vi "tag select action.vi"(8 "engine":refnum<data-value>, 10 "CtlRef":refnum<vi>, 11 "module editor":refnum<data-value>) -> (0 "error out":errorcluster)   [LabVIEW 2013, in "My Awesome Control Modules editor node.lvclass"]
uses:
  My Awesome Control Modules editor node.lvclass
  <vilib>/NI/Tag Bus Data Framework/control module/configuration/control module configuration.lvclass
  <vilib>/NI/Tag Bus/tag/tag descriptor.lvclass
  <vilib>/NI/Configuration Framework/serializable configuration/NISE_CEF_serializable configuration.lvclass
  <vilib>/NI/Tag Bus Data Framework/Configuration Editor/Classes/Engine Parent/Engine Parent Editor Node.lvclass
  <vilib>/NI/Module Execution Interface/Engine Configuration/engine configuration.lvclass
  <vilib>/NI/Tag Bus Data Framework/control module/editor node/control module editor.lvclass
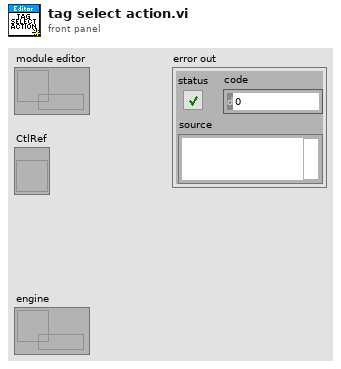
[diagram p1: front panel]
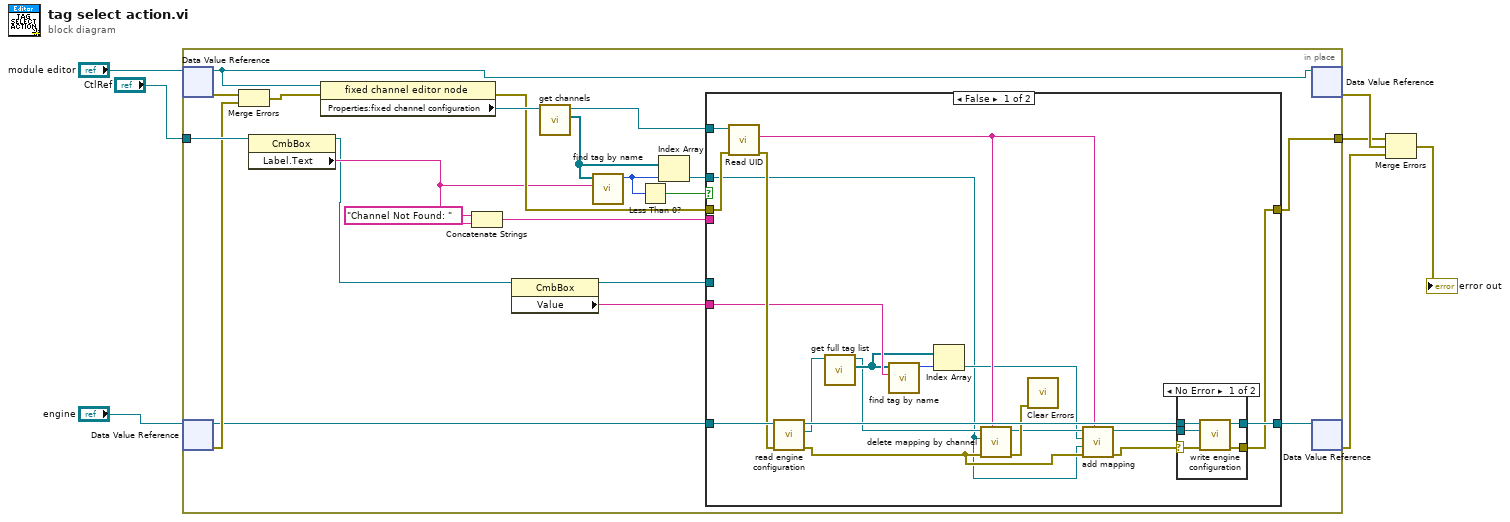
[diagram p0: block diagram]
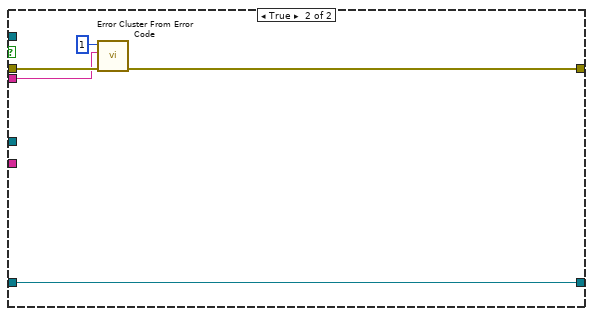
[diagram p3: hidden frame]
diagram:
  n1 = in-place {
    in-place-border: [w23] -> w2
    in-place-border: "CtlRef" -> [w21]
    n2 = in-place-dvr #1("module editor") -> (w13:refnum<class "control module editor.lvclass">, w28:errorcluster)
    n3 = in-place-dvr #2("engine") -> (w12:refnum<class "Engine Parent Editor Node.lvclass">, w15:errorcluster)
    n4 = Merge Errors(w28, w15) -> (w16:errorcluster)
    n5 = property class="CmbBox"(reference=w21) -> (reference out=w11:refnum<vi>, "Label.Text"=w20:string)  [unwired: 1 in, 1 out]
    n6 = property class="fixed channel editor node"(reference=w13, error in=w16) -> (error out=w22:errorcluster, "Properties:fixed channel configuration"=w27:refnum<class "control module configuration.lvclass">)  [unwired: 1 out]
    n7 = Concatenate Strings("Channel Not Found: " ("string"), w20) -> (w18:string)
    n8 = property class="CmbBox"(reference=w11) -> (reference out=w10:refnum<vi>, "Value"=w9:string)  [unwired: 1 in, 1 out]
    n9 = call-dynamic "get channels.vi"("fixed channel configuration in"=w27) -> ("channels"=w26:refnum<class "TBM channel.lvclass">[], "fixed channel configuration out"=w14:refnum<class "control module configuration.lvclass">)  [unwired: 9 in]
    n10 = call <vilib>:"find tag by name.vi"("name"=w20, "tags in"=w26) -> ("index"=w25:i32)  [unwired: 9 in]
    n11 = Less Than 0?(x=w25) -> (x < 0?=w24:bool)
    n12 = Index Array(array=w26, index=w25) -> (element=w17:refnum<class "TBM channel.lvclass">)
    n13 = case shown="False" w24 {
      tunnel: [w43 w59] -> w23
      tunnel: w22 -> [w47 w58]
      tunnel: w18 -> [_ w57]
      tunnel: w17 -> [w29 _]
      tunnel: w14 -> [w48 _]
      tunnel: w12 -> [w46 w56]
      tunnel: w10 -> [_ _]
      tunnel: w9 -> [w41 _]
      tunnel: [w44 w56] -> w8
      frame False {
        n14 = call <vilib>:"Read UID.vi"("error in"=w47, "configuration in"=w48) -> ("error out"=w45:errorcluster, "instance id"=w33:string)  [unwired: 7 in, 1 out]
        n15 = call <vilib>:"read engine configuration.vi"("error in"=w45, "Engine Parent Editor Node in"=w46) -> ("error out"=w35:errorcluster, "engine configuration"=w38:refnum<class "engine configuration.lvclass">, "Engine Parent Editor Node out"=w42:refnum<class "Engine Parent Editor Node.lvclass">)  [unwired: 7 in]
        n16 = call <vilib>:"get full tag list.vi"("engine configuration in"=w38) -> ("tag list"=w39:refnum<class "tag descriptor.lvclass">[], "engine configuration out"=w37:refnum<class "engine configuration.lvclass">)  [unwired: 9 in]
        n17 = call <vilib>:"find tag by name.vi"("name"=w41, "tags in"=w39) -> ("index"=w40:i32)  [unwired: 9 in]
        n18 = Index Array(array=w39, index=w40) -> (element=w30:refnum<class "tag descriptor.lvclass">)
        n19 = call <vilib>:"delete mapping by channel.vi"("owner ID"=w33, "error in"=w35, "channel"=w29, "engine configuration in"=w37) -> ("error out"=w36:errorcluster, "engine configuration out"=w34:refnum<class "engine configuration.lvclass">)  [unwired: 6 in]
        n20 = call <vilib>:"Clear Errors.vi"("error in (no error)"=w36) -> ()  [unwired: 5 in, 2 out]
        n21 = call <vilib>:"add mapping.vi"("owner ID"=w33, "error in"=w35, "channel"=w29, "tag descriptor"=w30, "engine configuration"=w34) -> ("error out"=w32:errorcluster, "engine configuration out"=w31:refnum<class "engine configuration.lvclass">)  [unwired: 5 in]
        n22 = case shown="No Error" w32 {
          selector: w32 -> [w52 w54]
          tunnel: [w53 w55] -> w44
          tunnel: [w51 w54] -> w43
          tunnel: w42 -> [w50 w55]
          tunnel: w31 -> [w49 _]
          frame No Error {
            n23 = call <vilib>:"write engine configuration.vi"("error in"=w52, "engine configuration"=w49, "Engine Parent Editor Node in"=w50) -> ("error out"=w51:errorcluster, "Engine Parent Editor Node out"=w53:refnum<class "Engine Parent Editor Node.lvclass">)  [unwired: 7 in]
          }
          frame Error {
          }
        }
      }
      frame True {
        n24 = call <vilib>:"Error Cluster From Error Code.vi"("error in (no error)"=w58, "error message (\"\")"=w57, "error code (0)"=1) -> ("error out"=w59:errorcluster)  [unwired: 6 in]
      }
    }
    n25 = in-place-dvr #1(w13) -> (w3:errorcluster)  [unwired: 1 out]
    n26 = in-place-dvr #2(w8) -> (w6:errorcluster)  [unwired: 1 out]
  }
  n27 = Merge Errors(w2, w3, w6) -> (→"error out":errorcluster)
